vi "PIFOC Settings.vi"() -> ()   [LabVIEW 2020]
uses:
  _Controls/PIFOC Settings.ctl
panel:
  in  "PIFOC Settings":T1
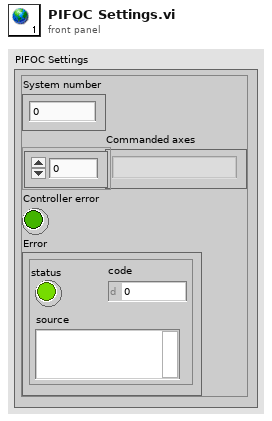
[diagram p1: front panel]
types:
  T1 = typedef "PIFOC Settings.ctl" = cluster{"System number":i32, "Commanded axes":string[], "Controller error":bool, "Error":errorcluster}
diagram:
